vi "Init Device.vi"(8 "error in (no error)":errorcluster, 11 "Ti2 in":refnum<class "Microscope.lvclass">) -> (0 "error out":errorcluster, 3 "Ti2 out":refnum<class "Microscope.lvclass">)   [LabVIEW 2018, in "Microscope.lvlib" / "Microscope.lvclass"]
uses:
  Microscope.lvclass
  Device/Device.lvclass
  ti2lv/ti2lv.lvlib
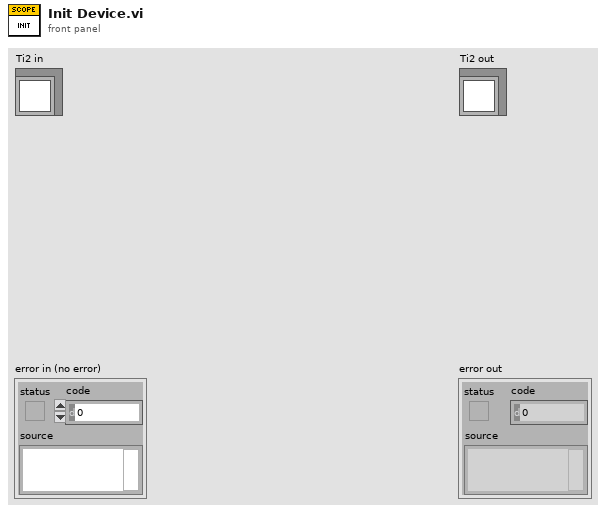
[diagram p1: front panel]
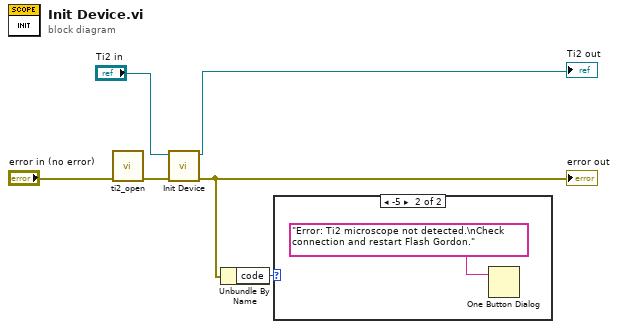
[diagram p0: block diagram]
diagram:
  n1 = call "ti2_open.vi"("error in (no error)"="error in (no error)") -> ("error out"=w3:errorcluster)  [unwired: 10 in]
  n2 = call-parent "Init Device.vi"("error in (no error)"=w3, "Device in"="Ti2 in") -> ("error out"=w2:errorcluster, "Device out"=→"Ti2 out":refnum<class "Microscope.lvclass">)  [unwired: 8 in]
  "error out" <- w2
  n3 = Unbundle By Name(w2) -> ("code"=w1:i32)
  n4 = case shown="-5" w1 {
    frame 0, Default {
    }
    frame -5 {
      n5 = One Button Dialog(message="Error: Ti2 microscope not detected.\nCheck connection and restart Flash Gordon.") -> ()  [unwired: 1 in, 1 out]
    }
  }
